vi "Teleop.vi"(10 "Match Info":T1={"Autonomous Elapsed Seconds"=0.0, "TeleOp Elapsed Seconds"=0.0, "Disabled Elapsed Seconds"=0.0, "Visited Autonomous"=FALSE, "Visited TeleOp"=FALSE, "Visited Disabled"=FALSE, "Autonomous Settings"={"Autonomous Style"=enum."Independent", "VI Refnum"=refnum}}, 11 "Call Context":T2) -> ()   [LabVIEW 2013]
doc: "This VI is called for each TeleOp packet received from the DS where the robot is not disabled. It is often used to read from the joysticks and update I/O or to update setpoints for timed control loops. It should complete and return within 20 milliseconds or it may miss DS packets."
uses:
  Robot Global Data.vi
  <vilib>/Rock Robotics/WPI/Solenoid/WPI_SolenoidValue.ctl
  <vilib>/Rock Robotics/WPI/Solenoid/Deprecated/WPI_SolenoidGetBool.vi
  <vilib>/Rock Robotics/WPI/Solenoid/WPI_SolenoidSetEnum.vi
  <vilib>/Rock Robotics/WPI/DriverStation/WPI_DriverStationMatch Info.ctl
  <vilib>/Rock Robotics/WPI/DriverStation/WPI_DriverStationDerivedRobotMode.ctl
panel:
  out "POT Value":dbl
  out "Numeric 1":dbl(slide) scale=0.0..100.0
  out "Boolean 2":bool
  out "Boolean 1":bool
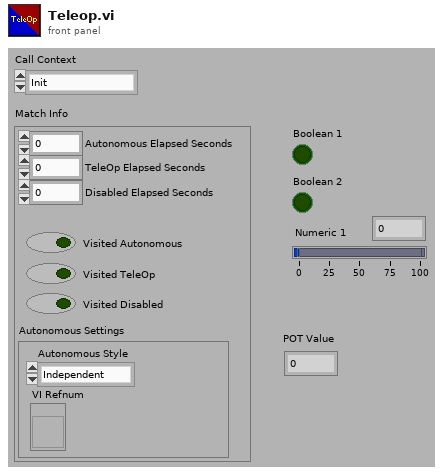
[diagram p1: front panel]
types:
  T1 = typedef "WPI_DriverStationMatch Info.ctl" = cluster{"Autonomous Elapsed Seconds":dbl, "TeleOp Elapsed Seconds":dbl, "Disabled Elapsed Seconds":dbl, "Visited Autonomous":bool, "Visited TeleOp":bool, "Visited Disabled":bool, "Autonomous Settings":cluster{"Autonomous Style":enum16{"Iterative", "Independent"}, "VI Refnum":refnum<vi>}}
  T2 = typedef "WPI_DriverStationDerivedRobotMode.ctl" = enum16{"Init", "Execute", "Stop"}
  T3 = typedef "WPI_JoystickDevRef.ctl" = cluster{"Device":T4}
  T4 = typedef "WPI_JoystickDeviceEnum.ctl" = enum16{"USB 1", "USB 2", "USB 3", "USB 4", "Kinect 1", "Kinect 2"}
  T5 = typedef "WPI_JoystickButtonState.ctl" = cluster{"Button 1":bool, "Button 2":bool, "Button 3":bool, "Button 4":bool, "Button 5":bool, "Button 6":bool, "Button 7":bool, "Button 8":bool, "Button 9":bool, "Button 10":bool, "Button 11":bool, "Button 12":bool}
  T6 = typedef "WPI_SolenoidDevRef.ctl" = cluster{"DevStatus":errorcluster, "Solenoid Module":T7, "Forward Solenoid Channel":T8, "Reverse Solenoid Channel":T8}
  T7 = typedef "FPGA_TypedefSolenoidModule.ctl" = enum16{"Solenoid Module 1", "Solenoid Module 2"}
  T8 = typedef "WPI_SolenoidChannel.ctl" = enum8{"Solenoid 1", "Solenoid 2", "Solenoid 3", "Solenoid 4", "Solenoid 5", "Solenoid 6", "Solenoid 7", "Solenoid 8", "Invalid"}
  T9 = typedef "WPI_AnalogChannelDevRef.ctl" = cluster{"DevStatus":errorcluster, "Analog Module":T10, "Analog Channel":T11}
  T10 = typedef "FPGA_TypedefAnalogModule.ctl" = enum16{"Analog Module 1", "Analog Module 2"}
  T11 = typedef "FPGA_AIChannel.ctl" = enum8{"AI 1", "AI 2", "AI 3", "AI 4", "AI 5", "AI 6", "AI 7", "AI 8", "Invalid"}
  T12 = typedef "WPI_DigitalInputDevRef.ctl" = cluster{"DevStatus":errorcluster, "DIO Channel":T13, "Digital Module":T14}
  T13 = typedef "FPGA_DIOChannel.ctl" = enum8{"DIO 1", "DIO 2", "DIO 3", "DIO 4", "DIO 5", "DIO 6", "DIO 7", "DIO 8", "DIO 9", "DIO 10", "DIO 11", "DIO 12", "DIO 13", "DIO 14", "Invalid"}
  T14 = typedef "FPGA_TypedefDigitalModule.ctl" = enum16{"Digital Module 1", "Digital Module 2"}
  T15 = typedef "WPI_MotorControlDeviceRef.ctl" = cluster{"DeviceStatus":errorcluster, "Type":enum16{"PWM", "CAN"}, "PWM":cluster{"Digital Module":T14, "PWM Channel":T16, "DeadBand":T17}, "CAN":cluster{"Device Number":u8, "Control Mode":T18, "Semaphore":T19, "Max Vout":dbl}, "Invert":bool, "TransformRef":T20, "InvTransformRef":T20}
  T16 = typedef "FPGA_DIOPWMChannel.ctl" = enum8{"PWM 1", "PWM 2", "PWM 3", "PWM 4", "PWM 5", "PWM 6", "PWM 7", "PWM 8", "PWM 9", "PWM 10", "Invalid"}
  T17 = typedef "WPI_PWMDeadband.ctl" = cluster{"Name":string, "maxPositivePwm":i32, "minPositivePwm":i32, "centerPwm":i32, "maxNegativePwm":i32, "minNegativePwm":i32, "angularRange":u16}
  T18 = typedef "WPI_CANJaguar_ControlMode.ctl" = enum8{"Percent VBus", "Current", "Speed", "Position", "Voltage"}
  T19 = typedef "Semaphore RefNum" = refnum<k1>
  T20 = typedef "WPI_PWMTransform_ConPane.ctl" = refnum<vi>
  T21 = typedef "WPI_RobotDriveDevRef.ctl" = cluster{"DevStatus":errorcluster, "Motors[]":T15[], "Square Inputs":bool, "Max Output":dbl, "Isochronous":bool}
  T22 = cluster{"axis 1 (x)":dbl, "axis 2 (y)":dbl, "axis 3 (throttle)":dbl, "axis 4":dbl, "axis 5":dbl, "axis 6":dbl}
  T23 = typedef "WPI_SolenoidValue.ctl" = enum16{"Off", "On", "Forward", "Reverse"}
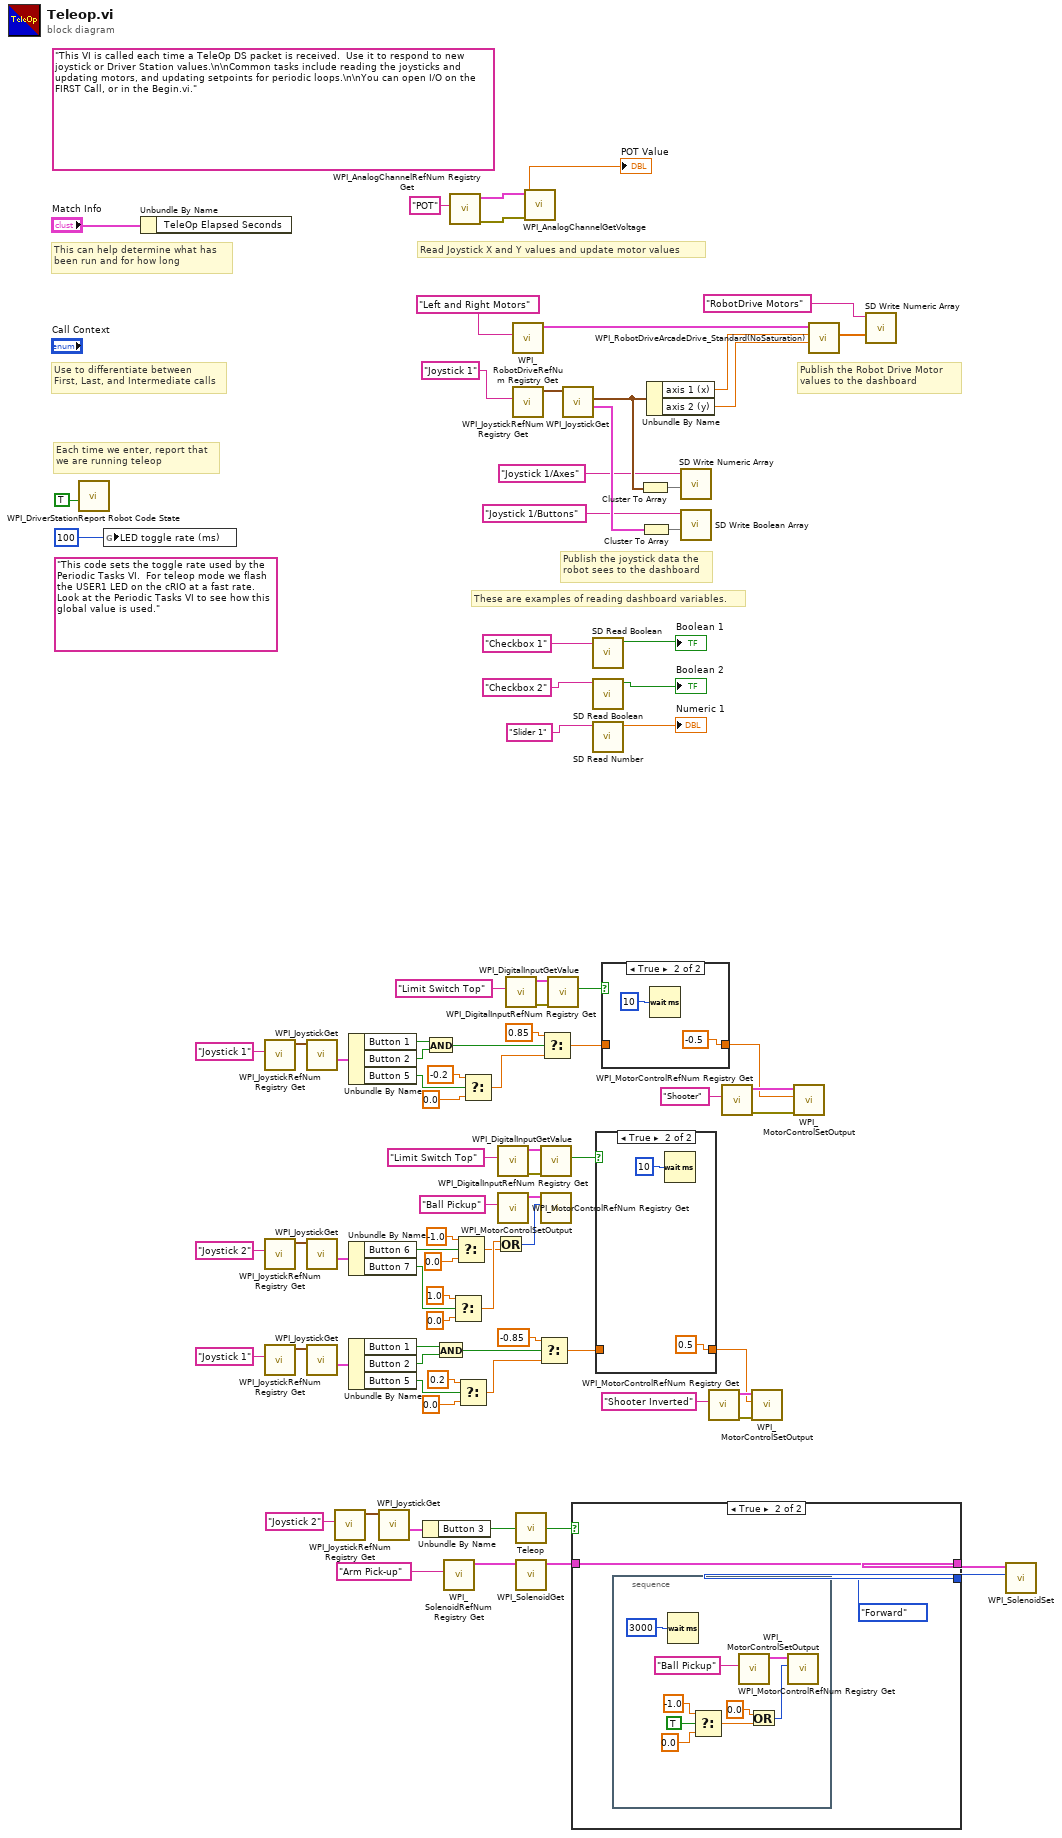
[diagram p0: block diagram]
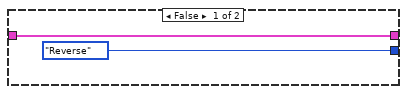
[diagram p4: hidden frame]
diagram:
  (unwired) "This code sets the toggle rate used by the Periodic Tasks VI.  For teleop mode we flash the USER1 LED on the cRIO at a fast rate.  Look at the Periodic Tasks VI to see how this global value is used."
  (unwired) "This VI is called each time a TeleOp DS packet is received.  Use it to respond to new joystick or Driver Station values.\n\nCommon tasks include reading the joysticks and updating motors, and updating setpoints for periodic loops.\n\nYou can open I/O on the FIRST Call, or in the Begin.vi."
  # "These are examples of reading dashboard variables."
  # "Publish the Robot Drive Motor\nvalues to the dashboard"
  # "Publish the joystick data the\nrobot sees to the dashboard"
  # "Each time we enter, report that\nwe are running teleop"
  # "Use to differentiate between\nFirst, Last, and Intermediate calls"
  # "This can help determine what has\nbeen run and for how long"
  # "Read Joystick X and Y values and update motor values"
  n1 = call <vilib>:"WPI_DriverStationReport Robot Code State.vi"("TeleOp"=TRUE ("Autonomous")) -> ()  [unwired: 10 in, 1 out]
  n2 = global write "Robot Global Data.vi" "LED toggle rate (ms)"(u32 100 ("LED ms toggle rate")) -> ()
  n3 = Unbundle By Name("Match Info") -> ()  [unwired: 1 out]
  n4 = call <vilib>:"WPI_JoystickRefNum Registry Get.vi"("refnum name"="Joystick 1") -> ("JoystickDevRef"=w67:T3)  [unwired: 9 in, 1 out]
  n5 = call <vilib>:"WPI_JoystickRefNum Registry Get.vi"("refnum name"="Joystick 2") -> ("JoystickDevRef"=w50:T3)  [unwired: 9 in, 1 out]
  n6 = call <vilib>:"WPI_JoystickRefNum Registry Get.vi"("refnum name"="Joystick 1") -> ("JoystickDevRef"=w60:T3)  [unwired: 9 in, 1 out]
  n7 = call <vilib>:"WPI_JoystickGet.vi"("JoystickDevRef"=w67) -> ("Buttons"=w66:T5)  [unwired: 4 in, 2 out]
  n8 = call <vilib>:"WPI_JoystickGet.vi"("JoystickDevRef"=w50) -> ("Buttons"=w51:T5)  [unwired: 4 in, 2 out]
  n9 = call <vilib>:"WPI_JoystickGet.vi"("JoystickDevRef"=w60) -> ("Buttons"=w61:T5)  [unwired: 4 in, 2 out]
  n10 = call <vilib>:"WPI_JoystickRefNum Registry Get.vi"("refnum name"="Joystick 2") -> ("JoystickDevRef"=w42:T3)  [unwired: 9 in, 1 out]
  n11 = Unbundle By Name(w66) -> ("Button 1"=w9:bool, "Button 2"=w8:bool, "Button 5"=w6:bool)
  n12 = Unbundle By Name(w51) -> ("Button 6"=w52:bool, "Button 7"=w48:bool)
  n13 = Unbundle By Name(w61) -> ("Button 1"=w10:bool, "Button 2"=w11:bool, "Button 5"=w7:bool)
  n14 = call <vilib>:"WPI_JoystickGet.vi"("JoystickDevRef"=w42) -> ("Buttons"=w41:T5)  [unwired: 4 in, 2 out]
  n15 = Unbundle By Name(w41) -> ("Button 3"=w20:bool)
  n16 = And(x=w9, y=w8) -> (x .and. y?=w35:bool)
  n17 = And(x=w10, y=w11) -> (x .and. y?=w62:bool)
  n18 = call <vilib>:"WPI_SolenoidRefNum Registry Get.vi"("refnum name"="Arm Pick-up") -> ("SolenoidDevRef"=w40:T6)  [unwired: 9 in, 1 out]
  n19 = call <vilib>:"WPI_AnalogChannelRefNum Registry Get.vi"("refnum name"="POT") -> ("error out"=w23:errorcluster, "AIDeviceRef"=w22:T9)  [unwired: 9 in]
  n20 = Select(t=1.0, s=w48, f=0.0) -> (s? t:f=w47:dbl)
  n21 = Select(t=-1.0, s=w52, f=0.0) -> (s? t:f=w46:dbl)
  n22 = Select(t=0.2, s=w7, f=0.0) -> (s? t:f=w12:dbl)
  n23 = Select(t=-0.2, s=w6, f=0.0) -> (s? t:f=w13:dbl)
  n24 = Or(x=w47, y=w46) -> (x .or. y?=w45:i32)
  n25 = call <vilib>:"WPI_DigitalInputRefNum Registry Get.vi"("refnum name"="Limit Switch Top") -> ("error out"=w28:errorcluster, "DigitalInputDevRef"=w29:T12)  [unwired: 9 in]
  n26 = call <vilib>:"WPI_MotorControlRefNum Registry Get.vi"("refnum name"="Ball Pickup") -> ("MotorControlDevRef"=w57:T15)  [unwired: 9 in, 1 out]
  n27 = call <vilib>:"WPI_DigitalInputRefNum Registry Get.vi"("refnum name"="Limit Switch Top") -> ("error out"=w33:errorcluster, "DigitalInputDevRef"=w32:T12)  [unwired: 9 in]
  n28 = call <vilib>:"WPI_RobotDriveRefNum Registry Get.vi"("refnum name"="Left and Right Motors") -> ("RobotDriveDevRef"=w89:T21)  [unwired: 1 in, 9 out]
  n29 = call <vilib>:"WPI_JoystickRefNum Registry Get.vi"("refnum name"="Joystick 1") -> ("JoystickDevRef"=w85:T3)  [unwired: 1 in, 9 out]
  n30 = call "Teleop.vi"("Input"=w20) -> ("Toggled Output"=w39:bool)
  n31 = call-poly <vilib>:"WPI_SolenoidGet.vi"("SolenoidDevRef"=w40) -> ("SolenoidDevRef"=w38:T6)  [unwired: 8 in, 2 out]
  n32 = call <vilib>:"WPI_AnalogChannelGetVoltage.vi"("error in (no error)"=w23, "AIDeviceRef"=w22) -> ("Voltage"=→"POT Value":dbl)  [unwired: 7 in, 2 out]
  n33 = Select(t=-0.85, s=w62, f=w12) -> (s? t:f=w25:dbl)
  n34 = call <vilib>:"WPI_DigitalInputGetValue.vi"("error in (no error)"=w28, "DigitalInputDevRef"=w29) -> ("Value"=w26:bool)  [unwired: 7 in, 2 out]
  n35 = call <vilib>:"WPI_MotorControlSetOutput.vi"("Output"=w45, "MotorControlDevRef"=w57) -> ()  [unwired: 7 in, 3 out]
  n36 = Select(t=0.85, s=w35, f=w13) -> (s? t:f=w30:dbl)
  n37 = call <vilib>:"WPI_DigitalInputGetValue.vi"("error in (no error)"=w33, "DigitalInputDevRef"=w32) -> ("Value"=w31:bool)  [unwired: 7 in, 2 out]
  n38 = call <vilib>:"WPI_JoystickGet.vi"("JoystickDevRef"=w85) -> ("Buttons"=w82:T5, "Axes"=w79:T22)  [unwired: 1 in, 4 out]
  n39 = case shown="True" w39 {
    tunnel: w38 -> [w93 w95]
    tunnel: [w93 w95] -> w37
    tunnel: [WPI_SolenoidValue."Reverse" ("Value") WPI_SolenoidValue."Forward" ("Value")] -> w36
    frame False {
    }
    frame True {
      n40 = stacked-sequence {
        frame #0 {
          n41 = Wait (ms)(milliseconds to wait=u32 3000) -> ()  [unwired: 1 out]
          n42 = Select(t=-1.0, s=TRUE, f=0.0) -> (s? t:f=w99:dbl)
          n43 = call <vilib>:"WPI_MotorControlRefNum Registry Get.vi"("refnum name"="Ball Pickup") -> ("MotorControlDevRef"=w102:T15)  [unwired: 9 in, 1 out]
          n44 = Or(x=0.0, y=w99) -> (x .or. y?=w98:i32)
          n45 = call <vilib>:"WPI_MotorControlSetOutput.vi"("Output"=w98, "MotorControlDevRef"=w102) -> ()  [unwired: 7 in, 3 out]
        }
      }
    }
  }
  n46 = call <vilib>:"SD Read Boolean.vi"("Name"="Checkbox 1" ("refnum name")) -> ("Boolean"=→"Boolean 1":bool)  [unwired: 8 in, 2 out]
  n47 = call <vilib>:"SD Read Boolean.vi"("Name"="Checkbox 2" ("refnum name")) -> ("Boolean"=→"Boolean 2":bool)  [unwired: 8 in, 2 out]
  n48 = call <vilib>:"SD Read Number.vi"("Name"="Slider 1" ("refnum name")) -> ("Numeric"=→"Numeric 1":dbl)  [unwired: 8 in, 2 out]
  n49 = case shown="True" w26 {
    tunnel: [w105 0.5 ("f")] -> w1
    tunnel: w25 -> [w105 _]
    frame False {
    }
    frame True {
      n50 = Wait (ms)(milliseconds to wait=u32 10) -> ()  [unwired: 1 out]
    }
  }
  n51 = case shown="True" w31 {
    tunnel: [w108 -0.5 ("f")] -> w2
    tunnel: w30 -> [w108 _]
    frame False {
    }
    frame True {
      n52 = Wait (ms)(milliseconds to wait=u32 10) -> ()  [unwired: 1 out]
    }
  }
  n53 = Cluster To Array(cluster=w79) -> (array=w78:dbl[])
  n54 = Cluster To Array(cluster=w82) -> (array=w81:bool[])
  n55 = Unbundle By Name(w79) -> ("axis 1 (x)"=w88:dbl, "axis 2 (y)"=w87:dbl)
  n56 = call <vilib>:"SD Write Numeric Array.vi"("Numeric Array"=w78, "Name"="Joystick 1/Axes") -> ()  [unwired: 8 in, 2 out]
  n57 = call <vilib>:"SD Write Boolean Array.vi"("Boolean Array"=w81, "Name"="Joystick 1/Buttons") -> ()  [unwired: 8 in, 2 out]
  n58 = call <vilib>:"WPI_MotorControlRefNum Registry Get.vi"("refnum name"="Shooter Inverted") -> ("error out"=w4:errorcluster, "MotorControlDevRef"=w5:T15)  [unwired: 9 in]
  n59 = call <vilib>:"WPI_MotorControlRefNum Registry Get.vi"("refnum name"="Shooter") -> ("error out"=w64:errorcluster, "MotorControlDevRef"=w63:T15)  [unwired: 9 in]
  n60 = call <vilib>:"WPI_MotorControlSetOutput.vi"("error in (no error)"=w4, "Output"=w1, "MotorControlDevRef"=w5) -> ()  [unwired: 6 in, 3 out]
  n61 = call <vilib>:"WPI_MotorControlSetOutput.vi"("error in (no error)"=w64, "Output"=w2, "MotorControlDevRef"=w63) -> ()  [unwired: 6 in, 3 out]
  n62 = call <vilib>:"WPI_RobotDriveArcadeDrive_Standard(NoSaturation).vi"("Y axis value"=w87, "X axis value"=w88, "RobotDriveDevRef"=w89) -> ("Motor Values"=w75:dbl[])  [unwired: 1 in, 7 out]
  n63 = call <vilib>:"SD Write Numeric Array.vi"("Numeric Array"=w75, "Name"="RobotDrive Motors") -> ()  [unwired: 8 in, 2 out]
  n64 = call-poly <vilib>:"WPI_SolenoidSet.vi"("Value"=w36, "SolenoidDevRef"=w37) -> ()  [unwired: 8 in, 2 out]
